vi "enable error reporting.vi"(8 "error in":errorcluster, 9 "tag":string, 10 "module ID":string, 11 "Standard Engine Configuration in":refnum<class "Standard Engine Configuration.lvclass">) -> (0 "error out":errorcluster, 3 "Standard Engine Configuration out":refnum<class "Standard Engine Configuration.lvclass">)   [LabVIEW 2013, in "Standard Engine Configuration.lvclass"]
uses:
  Standard Engine Configuration.lvclass
  <vilib>/NI/Tag Bus Module Framework/channel/channel classification.ctl
  <vilib>/NI/Tag Bus/tag/Data Type.ctl
  <vilib>/NI/Tag Bus Module Framework/root configuration/TBM configuration.lvclass/TBM configuration.ctl
  Standard Engine Configuration.lvclass/Standard Engine Configuration.ctl
  <vilib>/NI/Tag Bus Module Framework/root configuration/create GUID.vi
  <vilib>/NI/Module Execution Interface/Engine Configuration/engine configuration.lvclass
  <vilib>/NI/Tag Bus Module Framework/root configuration/TBM configuration.lvclass
  <vilib>/NI/Tag Bus Module Framework/channel/TBM channel.lvclass
  <vilib>/NI/Tag Bus/tag/tag descriptor.lvclass
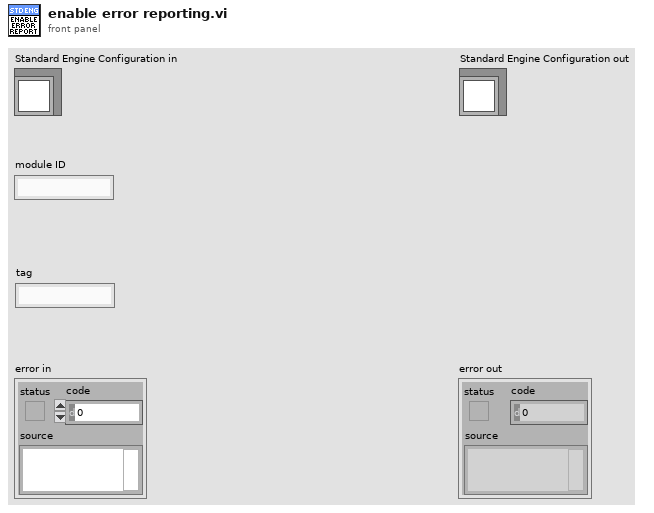
[diagram p1: front panel]
types:
  T1 = typedef "tag bus.lvlib/tag descriptor.lvclass/Data Type.ctl" = enum16{"Double", "Single", "I64", "I32", "I16", "I8", "U64", "U32", "U16", "U8", "Boolean", "String", "Array of Double", "Array of Single", "Array of I64", "Array of I32", "Array of I16", "Array of I8", "Array of U64", "Array of U32", "Array of U16", "Array of U8", "Array of Boolean", "Array of String"}
  T2 = typedef "TBM channel.lvclass/channel classification.ctl" = enum16{"input data", "output data", "processing parameter", "processing result"}
  T3 = typedef "Standard Engine Configuration.lvclass/Module Specific Configuration.ctl" = cluster{"Module ID":string, "Module Decimation":T4, "Module Error Configuration":T5, "execution order priority":i32, "async?":bool, "error tag":string}
  T4 = typedef "Standard Engine Configuration.lvclass/Module Decimation.ctl" = cluster{"Decimation":u16, "Offset":u16}
  T5 = typedef "Standard Engine Configuration.lvclass/Module Error Configuration.ctl" = cluster{"Module Error Configuration":T6[]}
  T6 = typedef "Standard Engine Configuration.lvclass/Error Actions By Category.ctl" = cluster{"error classification":T7, "Error Actions":T8[]}
  T7 = typedef "TBM module execution interface.lvclass/error classification.ctl" = enum16{"unknown", "none", "trivial", "recoverable", "critical"}
  T8 = typedef "Standard Engine Configuration.lvclass/Error Actions.ctl" = enum16{"Clear", "Notify", "Stop Component", "Stop Engine", "Safe State", "Attempt Recovery"}
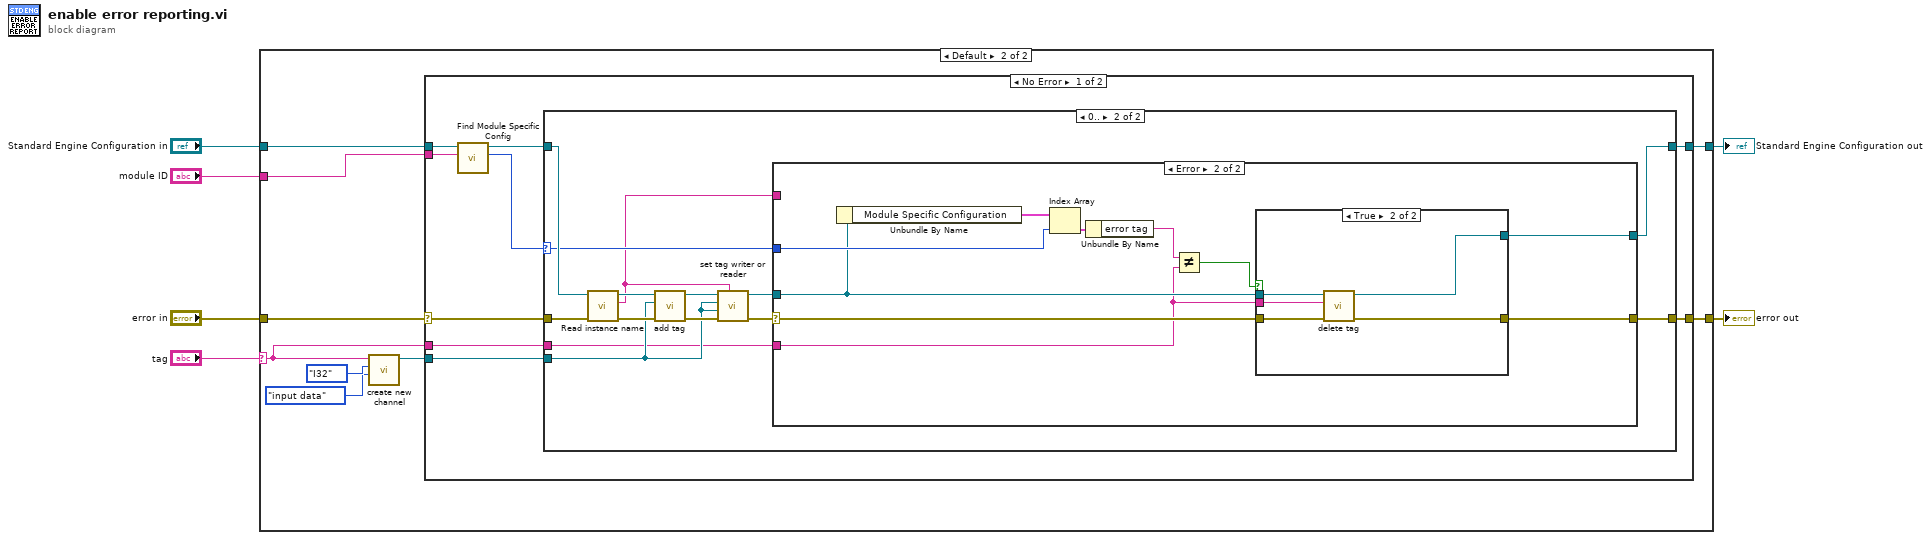
[diagram p0: block diagram]
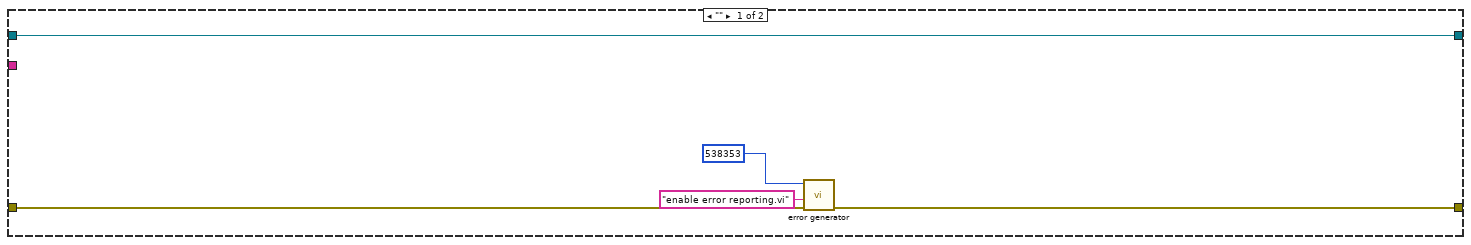
[diagram p2: hidden frame]
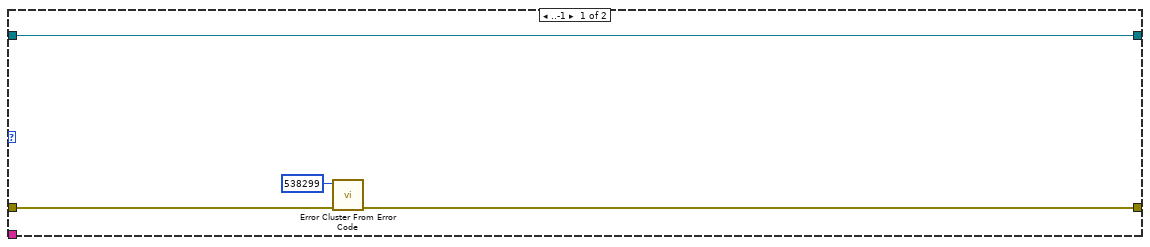
[diagram p3: hidden frame]
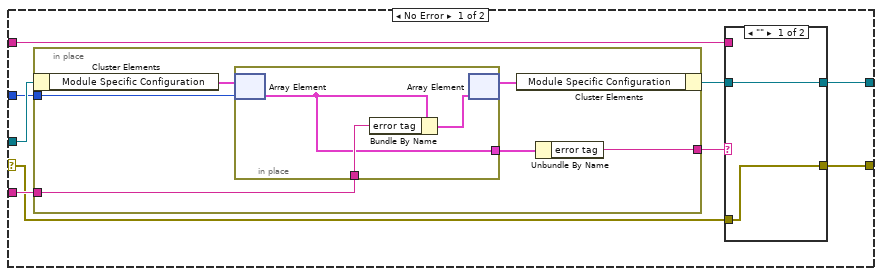
[diagram p4: hidden frame]
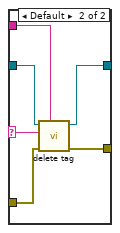
[diagram p5: hidden frame]
diagram:
  n1 = case shown="Default" "tag" {
    selector: "tag" -> [_ w12]
    tunnel: "Standard Engine Configuration in" -> [w11 w20]
    tunnel: "module ID" -> [_ w19]
    tunnel: "error in" -> [w10 w18]
    tunnel: [w11 w17] -> w3
    tunnel: [w9 w16] -> w2
    frame "" {
      n2 = call <vilib>:"error generator.vi"("error in"=w10, "source"="enable error reporting.vi", "error code (0)"=538353) -> ("error out"=w9:errorcluster)  [unwired: 8 in]
    }
    frame Default {
      n3 = call <vilib>:"create new channel.vi"("channel classification"=channel_classification."input data", "data type"=Data_Type."I32", "channel name"=w12) -> ("channel"=w15:refnum<class "TBM channel.lvclass">)  [unwired: 8 in]
      n4 = case shown="No Error" w18 {
        selector: w18 -> [w25 w92]
        tunnel: w20 -> [w29 w91]
        tunnel: w19 -> [w28 _]
        tunnel: [w23 w91] -> w17
        tunnel: [w24 w92] -> w16
        tunnel: w15 -> [w22 _]
        tunnel: w12 -> [w21 _]
        frame No Error {
          n5 = call "Find Module Specific Config.vi"("Module ID"=w28, "Standard Engine Repo Data in"=w29) -> ("Index"=w26:i32, "Standard Engine Repo Data out"=w27:refnum<class "Standard Engine Configuration.lvclass">)  [unwired: 8 in]
          n6 = case shown="0.." w26 {
            selector: w26 -> [_ w37]
            tunnel: w27 -> [w33 w43]
            tunnel: w25 -> [w32 w47]
            tunnel: [w31 w38] -> w24
            tunnel: [w33 w39] -> w23
            tunnel: w22 -> [_ w36]
            tunnel: w21 -> [_ w35]
            frame ..-1 {
              n7 = call <vilib>:"Error Cluster From Error Code.vi"("error in (no error)"=w32, "error code (0)"=538299) -> ("error out"=w31:errorcluster)  [unwired: 7 in]
            }
            frame 0.. {
              n8 = call <vilib>:"Read instance name.vi"("error in"=w47, "configuration in"=w43) -> ("error out"=w44:errorcluster, "instance id"=w34:string, "configuration out"=w42:refnum<class "Standard Engine Configuration.lvclass">)  [unwired: 7 in]
              n9 = call <vilib>:"add tag.vi"("error in"=w44, "tag descriptor"=w36, "engine configuration in"=w42) -> ("error out"=w46:errorcluster, "engine configuration out"=w45:refnum<class "Standard Engine Configuration.lvclass">)  [unwired: 7 in]
              n10 = call <vilib>:"set tag writer or reader.vi"("module GUID"=w34, "error in"=w46, "channel"=w36, "tag descriptor"=w36, "engine configuration in"=w45) -> ("error out"=w41:errorcluster, "engine configuration out"=w40:refnum<class "Standard Engine Configuration.lvclass">)  [unwired: 5 in]
              n11 = case shown="Error" w41 {
                selector: w41 -> [w50 w78]
                tunnel: w40 -> [w56 w79]
                tunnel: [w52 w76] -> w39
                tunnel: [w51 w77] -> w38
                tunnel: w37 -> [w55 w82]
                tunnel: w35 -> [w54 w75]
                tunnel: w34 -> [w49 _]
                frame No Error {
                  n12 = in-place {
                    in-place-border: w55 -> [w68]
                    in-place-border: w54 -> [w67]
                    in-place-border: [w65] -> w48
                    n13 = in-place-cluster #1(w56) -> ("Module Specific Configuration"=w70:T3[])
                    n14 = in-place {
                      in-place-border: w67 -> [w72]
                      in-place-border: [w71] -> w66
                      n15 = in-place-array #2(w70, w68) -> (w71:T3)
                      n16 = Bundle By Name(cluster=w71, "error tag"=w72) -> (w73:T3)
                      n17 = in-place-array #2(w73) -> (w69:T3[])  [unwired: 1 out]
                    }
                    n18 = in-place-cluster #1("Module Specific Configuration"=w69) -> (w53:refnum<class "Standard Engine Configuration.lvclass">)
                    n19 = Unbundle By Name(w66) -> ("error tag"=w65:string)
                  }
                  n20 = case shown="\"\"" w48 {
                    selector: w48 -> [_ w59]
                    tunnel: w53 -> [w58 w64]
                    tunnel: [w58 w63] -> w52
                    tunnel: [w57 w62] -> w51
                    tunnel: w50 -> [w57 w61]
                    tunnel: w49 -> [_ w60]
                    frame "" {
                    }
                    frame Default {
                      n21 = call <vilib>:"delete tag.vi"("owner ID"=w60, "error in"=w61, "tag name"=w59, "engine configuration in"=w64) -> ("error out"=w62:errorcluster, "engine configuration out"=w63:refnum<class "Standard Engine Configuration.lvclass">)  [unwired: 6 in]
                    }
                  }
                }
                frame Error {
                  n22 = Unbundle By Name(w79) -> ("Module Specific Configuration"=w83:T3[])
                  n23 = Index Array(array=w83, index=w82) -> (element=w81:T3)
                  n24 = Unbundle By Name(w81) -> ("error tag"=w80:string)
                  n25 = Not Equal?(x=w80, y=w75) -> (x != y?=w74:bool)
                  n26 = case shown="True" w74 {
                    tunnel: w79 -> [w85 w90]
                    tunnel: w78 -> [w84 w89]
                    tunnel: [w84 w88] -> w77
                    tunnel: [w85 w87] -> w76
                    tunnel: w75 -> [_ w86]
                    frame False {
                    }
                    frame True {
                      n27 = call <vilib>:"delete tag.vi"("error in"=w89, "tag name"=w86, "engine configuration in"=w90) -> ("error out"=w88:errorcluster, "engine configuration out"=w87:refnum<class "Standard Engine Configuration.lvclass">)  [unwired: 7 in]
                    }
                  }
                }
              }
            }
          }
        }
        frame Error {
        }
      }
    }
  }
  "error out" <- w2
  "Standard Engine Configuration out" <- w3
